vi "Sending Modulated Audio.vi"() -> ()   [LabVIEW 2019]
doc: "This application reads the selected audio file from its media storage. The audio is outputed through the Emona Communications Board for its modulation. After being modulated, the signal is inputed once again into the application. The modulated signal is now displayed through the Modulated Signal Graph and also is being sent to the other target by communicating with a TCP protocol."
uses:
  <vilib>/myRIO/Instrument Drivers/Onboard IO/AI Continuous/typedefs/AI Continuous Reference.ctl
  <vilib>/myRIO/Common/Instrument Driver Framework/Utilities/typedefs/myRIO Generic Hardware Reference.ctl
  <vilib>/myRIO/Common/Instrument Driver Framework/Utilities/typedefs/Hardware Version Enum.ctl
  <vilib>/myRIO/Common/Instrument Driver Framework/Utilities/typedefs/myRIO v1.0 Reference.ctl
  <vilib>/myRIO/Common/Instrument Driver Framework/Utilities/typedefs/Generic FPGA Reference.ctl
  <vilib>/myRIO/Common/Instrument Driver Framework/ELVIS III v1.0/AI Continuous/typedefs/AI Continuous Channels List.ctl
  <vilib>/myRIO/Common/Instrument Driver Framework/ELVIS III v1.0/AI Continuous/typedefs/ELVIS III v1.0 AI Continuous Channels Enum.ctl
  <vilib>/myRIO/Common/Instrument Driver Framework/Utilities/typedefs/Analog Scaling Constants.ctl
  <vilib>/userDefined/High Color/nirio_resource_hc.ctl
  <vilib>/myRIO/Instrument Drivers/Onboard IO/AO Continuous/typedefs/AO Continuous Reference.ctl
  <vilib>/myRIO/Common/Instrument Driver Framework/ELVIS III v1.0/AO Continuous/typedefs/AO Continuous Channels List.ctl
  <vilib>/myRIO/Common/Instrument Driver Framework/ELVIS III v1.0/AO Continuous/typedefs/ELVIS III v1.0 AO Continuous Channels Enum.ctl
  <vilib>/myRIO/Common/Instrument Driver Framework/ELVIS III v1.0/AO Continuous/typedefs/AO Continuous Channel Info.ctl
  <vilib>/myRIO/Instrument Drivers/Onboard IO/AO/typedefs/AO Reference.ctl
  <vilib>/myRIO/Common/Instrument Driver Framework/myRIO v1.0/AO/typedefs/AO Channels List.ctl
  <vilib>/myRIO/Common/Instrument Driver Framework/myRIO v1.0/AO/typedefs/AO Channels Enum.ctl
  <vilib>/myRIO/Common/Instrument Driver Framework/Utilities/typedefs/Analog Scaling Constants List.ctl
  <vilib>/myRIO/Common/Instrument Driver Framework/ELVIS III v1.0/AI Continuous/vis/ELVIS III v1.1 Open AI (Continuous).vi
  <vilib>/myRIO/Common/Instrument Driver Framework/ELVIS III v1.0/AO Continuous/vis/ELVIS III v1.1 Open AO (Continuous).vi
  <vilib>/myRIO/Common/Instrument Driver Framework/ELVIS III v1.0/AO/vis/ELVIS III v1.1 Open AO.vi
  <vilib>/myRIO/Common/Instrument Driver Framework/Utilities/vis/Validate Channels.vi
  <vilib>/myRIO/Common/Instrument Driver Framework/ELVIS III v1.0/AI Continuous/vis/ELVIS III v1.0 Reserve AI Continuous.vi
  <vilib>/myRIO/Common/Instrument Driver Framework/ELVIS III v1.0/AO Continuous/vis/ELVIS III v1.0 Reserve AO Continuous.vi
  <vilib>/myRIO/Common/Instrument Driver Framework/ELVIS III v1.0/AO/vis/ELVIS III v1.0 Reserve AO.vi
  <vilib>/myRIO/Common/Instrument Driver Framework/ELVIS III v1.0/AO Continuous/vis/ELVIS III v1.1 Close AO Continuous.vi
  <vilib>/myRIO/Common/Instrument Driver Framework/ELVIS III v1.0/AO/vis/ELVIS III v1.0 Close AO.vi
  <vilib>/myRIO/Common/Instrument Driver Framework/ELVIS III v1.0/AI Continuous/vis/ELVIS III v1.0 Close AI Continuous.vi
  <vilib>/myRIO/Common/Instrument Driver Framework/myRIO v1.0/UART/vis/myRIO v1.0 Close UART.vi
  <vilib>/myRIO/Common/Instrument Driver Framework/ELVIS III v1.0/AI Continuous/vis/ELVIS III v1.0 Build MUX Configuration AI Continuous.vi
  <vilib>/myRIO/Common/Instrument Driver Framework/ELVIS III v1.0/AO Continuous/vis/ELVIS III v1.0 Build MUX Configuration AO Continuous.vi
  <vilib>/myRIO/Common/Instrument Driver Framework/ELVIS III v1.0/AO/vis/ELVIS III v1.0 Build MUX Configuration AO.vi
  <vilib>/myRIO/Common/Instrument Driver Framework/ELVIS III v1.0/AO Continuous/vis/ELVIS III v1.0 Unreserve AO Continuous.vi
  <vilib>/myRIO/Common/Instrument Driver Framework/ELVIS III v1.0/AO/vis/ELVIS III v1.0 Unreserve AO.vi
  <vilib>/myRIO/Common/Instrument Driver Framework/ELVIS III v1.0/AI Continuous/vis/ELVIS III v1.0 Unreserve AI Continuous.vi
  <vilib>/Utility/VariantDataType/GetNumericInfo.vi
  <vilib>/Utility/error.llb/Error Cluster From Error Code.vi
  <vilib>/myRIO/Common/Instrument Driver Framework/ELVIS III v1.0/ELVIS III v1.1 Open.vi
  <vilib>/myRIO/Common/Instrument Driver Framework/ELVIS III v1.0/Resource Manager/vis/ELVIS III v1.0 Reserve Channel List.vi
  <vilib>/myRIO/Common/Instrument Driver Framework/myRIO v1.0/myRIO v1.0 Close.vi
  <vilib>/myRIO/Common/Instrument Driver Framework/ELVIS III v1.0/Resource Manager/vis/ELVIS III v1.0 Configure DMAs.vi
  <vilib>/myRIO/Common/Instrument Driver Framework/ELVIS III v1.0/AO Continuous/vis/ELVIS III v1.1 Stop AO Continuous.vi
  <vilib>/myRIO/Common/Instrument Driver Framework/ELVIS III v1.0/Resource Manager/vis/ELVIS III v1.0 Coerce AI Scaling.vi
  <vilib>/myRIO/Common/Instrument Driver Framework/ELVIS III v1.0/AI Continuous/vis/ELVIS III v1.1 Stop AI Continuous.vi
  <vilib>/myRIO/Common/Instrument Driver Framework/ELVIS III v1.0/AI Continuous/vis/ELVIS III v1.1 Start AI Continuous.vi
  <vilib>/myRIO/Common/Instrument Driver Framework/ELVIS III v1.0/AO Continuous/vis/ELVIS III v1.0 AO Continuous Write.vi
  <vilib>/myRIO/Common/Instrument Driver Framework/ELVIS III v1.0/AO/vis/ELVIS III v1.0 Write AO.vi
  <vilib>/myRIO/Common/Instrument Driver Framework/ELVIS III v1.0/AO Continuous/vis/ELVIS III v1.1 Start AO Continuous.vi
  <vilib>/myRIO/Common/Instrument Driver Framework/ELVIS III v1.0/AI Continuous/vis/ELVIS III v1.0 AI Continuous Read.vi
  <vilib>/myRIO/Common/Instrument Driver Framework/ELVIS III v1.0/Resource Manager/vis/ELVIS III v1.0 Unreserve Channel List.vi
  <vilib>/myRIO/Common/Instrument Driver Framework/Utilities/vis/FPGA Ref Manager.vi
  <vilib>/myRIO/Common/Instrument Driver Framework/ELVIS III v1.0/ELVIS III v1.0 Reset FPGA.vi
  <vilib>/myRIO/Common/Instrument Driver Framework/myRIO v1.0/IRQ/vis/myRIO v1.0 IRQ Info FGV.vi
  <vilib>/myRIO/Common/Instrument Driver Framework/myRIO v1.0/IRQ/vis/myRIO v1.0 Timer IRQ Info FGV.vi
  <vilib>/myRIO/Common/Instrument Driver Framework/myRIO v1.0/IRQ/vis/myRIO v1.0 ISR Agent.vi
  <vilib>/myRIO/Instrument Drivers/Utilities/vis/Reset Index.vi
  <vilib>/myRIO/Common/Instrument Driver Framework/myRIO v1.0/Resource Manager/vis/myRIO v1.0 Block Write Resource Manager.vi
  <vilib>/myRIO/Instrument Drivers/Onboard IO/AO/vis/myRIO AO Open.xnode
  <vilib>/myRIO/Instrument Drivers/Onboard IO/AO Continuous/vis/myRIO AO Continuous Open.xnode
  <vilib>/myRIO/Instrument Drivers/Onboard IO/AI Continuous/vis/myRIO AI Continuous Open.xnode
  <vilib>/myRIO/Instrument Drivers/Utilities/Utilities.lvlib
  <vilib>/myRIO/Instrument Drivers/Onboard IO/AO/AO.lvlib
  <vilib>/myRIO/Instrument Drivers/Onboard IO/AO Continuous/AO Continuous.lvlib
  <vilib>/myRIO/Instrument Drivers/Onboard IO/AI Continuous/AI Continuous.lvlib
panel:
  in  "Stop":bool
  in  "Select Audio":u16(ring) items=["ABBA- Dancing Queen.mp3", "Frank Sinatra - Fly Me To The Moon.mp3", "Gotye - Somebody That I Used To Know.mp3", "Mozart - Eine Kleine Nachtmusik.mp3"]
  in  "Address":string caption="Demodulator IP Address"
  out "Message":dbl[](graph) caption="Message History"
  in  "Offset":dbl=2.0
  out "Modulated Signal":dbl[](graph)
  out "error out":errorcluster
  in  "LocalStop":bool
  # "Sending and Modulating Audio"
  # "Explanation:\nThis application reads the selected audio file from its media storage. The audio is outputed through the Emona Communications Board for its modulation. After being modulated, the signal is inputed once again into the application. The modulated signal is now displayed through the Modulated Signal Graph and also is being sent to the other target by communicating with a TCP protocol.\n \nInstructions:\nAlways run the Receiving Modulated Audio VI before running this one. Remember to introduce the Demodulator IP Address into the control below. Check the instructions on the other VI for more information."
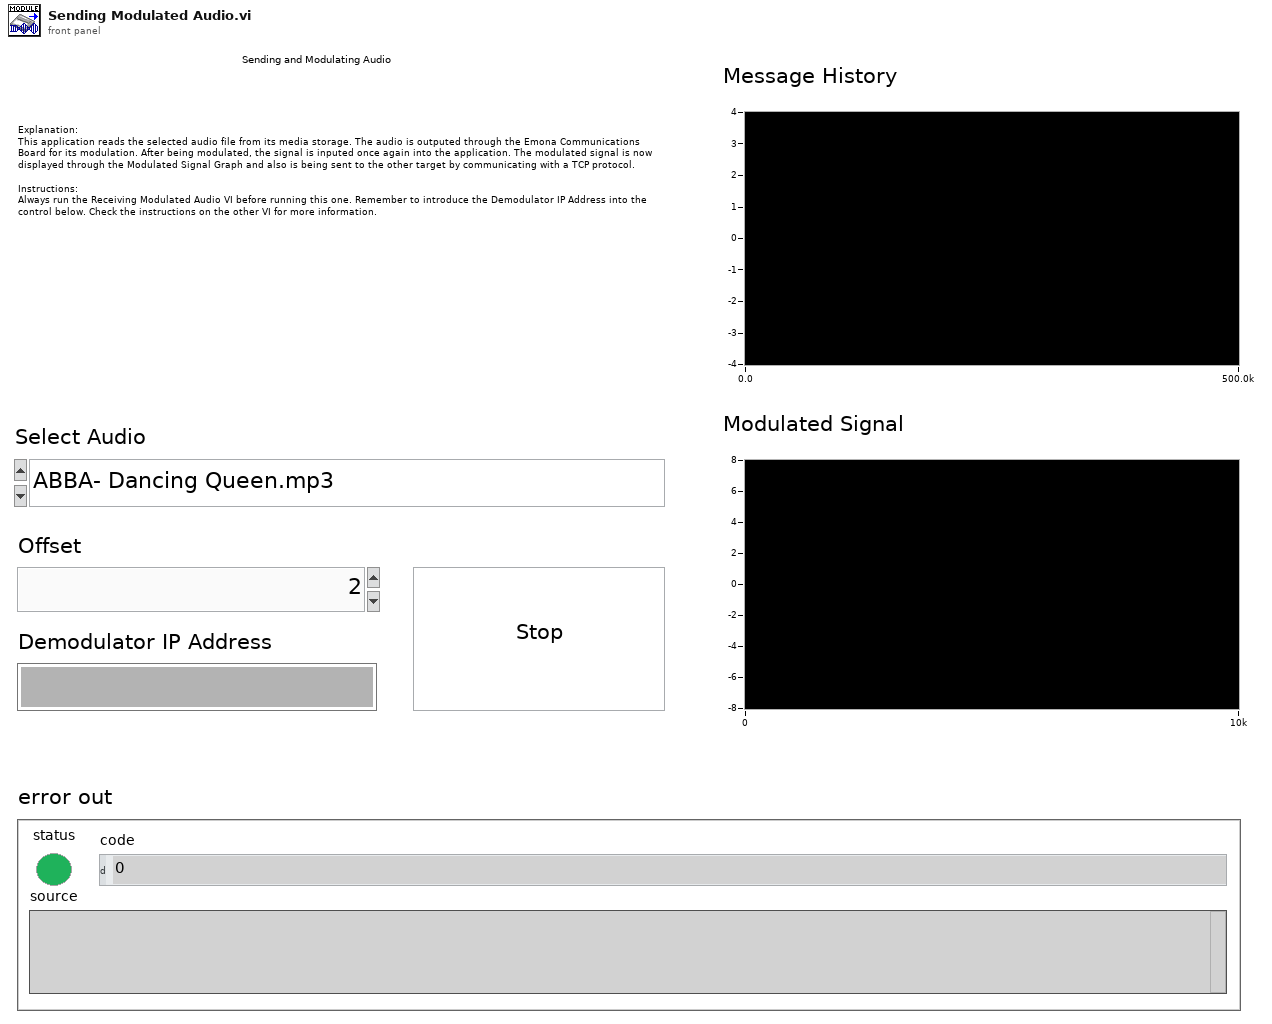
[diagram p1: front panel]
types:
  T1 = enum16{"open", "replace", "create", "open or create", "replace or create", "replace or create with confirmation"}
  T2 = typedef "AI Continuous.lvlib/AI Continuous Reference.ctl" = cluster{"myRIO Reference":T3, "AI (Continuous) Channels List":T7, "AI (Continuous) Scaling Constants List":T9[], "Bank Count":u8[]}
  T3 = typedef "myRIO Generic Hardware Reference.ctl" = cluster{"myRIO Model":T4, "myRIO Hardware Reference":T5}
  T4 = typedef "Hardware Version Enum.ctl" = enum16{"Unknown", "myRIO-1900", "myRIO-1950", "roboRIO", "NI ELVIS RIO CM", "ELVIS III"}
  T5 = typedef "myRIO v1.0 Reference.ctl" = cluster{"Generic FPGA Reference":T6, "Allow multiple opens":bool}
  T6 = typedef "Generic FPGA Reference.ctl" = refnum<k20>
  T7 = typedef "AI Continuous Channels List.ctl" = T8[]
  T8 = typedef "ELVIS III v1.0 AI Continuous Channels Enum.ctl" = enum16{"Not Connected", "A/AI0 (Continuous)", "A/AI1 (Continuous)", "A/AI2 (Continuous)", "A/AI3 (Continuous)", "A/AI4 (Continuous)", "A/AI5 (Continuous)", "A/AI6 (Continuous)", "A/AI7 (Continuous)", "A/AI0 (DIFF Continuous)", "A/AI1 (DIFF Continuous)", "A/AI2 (DIFF Continuous)", "A/AI3 (DIFF Continuous)", "B/AI0 (Continuous)", "B/AI1 (Continuous)", "B/AI2 (Continuous)", "B/AI3 (Continuous)", "B/AI4 (Continuous)", "B/AI5 (Continuous)", "B/AI6 (Continuous)", "B/AI7 (Continuous)", "B/AI0 (DIFF Continuous)", "B/AI1 (DIFF Continuous)", "B/AI2 (DIFF Continuous)", "B/AI3 (DIFF Continuous)"}
  T9 = typedef "Analog Scaling Constants.ctl" = cluster{"LSB Weight (Volts)":dbl, "Offset (Volts)":dbl, "Signed?":bool}
  T10 = typedef "AO Continuous.lvlib/AO Continuous Reference.ctl" = cluster{"myRIO Reference":T3, "AO (Continuous) Channels List":T11, "Channel Info":T13}
  T11 = typedef "AO Continuous Channels List.ctl" = T12[]
  T12 = typedef "ELVIS III v1.0 AO Continuous Channels Enum.ctl" = enum16{"Not Connected", "A/AO0 (Continuous)", "A/AO1 (Continuous)", "B/AO0 (Continuous)", "B/AO1 (Continuous)"}
  T13 = typedef "AO Continuous Channel Info.ctl" = cluster{"Channel Bitmask":u8[], "Channel Index":i32[], "Channel Number":u8}
  T14 = typedef "AO.lvlib/AO Reference.ctl" = cluster{"myRIO Reference":T3, "AO Channel List":T15, "AO Scaling Constant List":T17}
  T15 = typedef "AO Channels List.ctl" = T16[]
  T16 = typedef "AO Channels Enum.ctl" = enum16{"Not Connected", "AudioOut/Left", "AudioOut/Right", "C/AO0", "C/AO1", "A/AO0", "A/AO1", "B/AO0", "B/AO1"}
  T17 = typedef "Analog Scaling Constants List.ctl" = T9[]
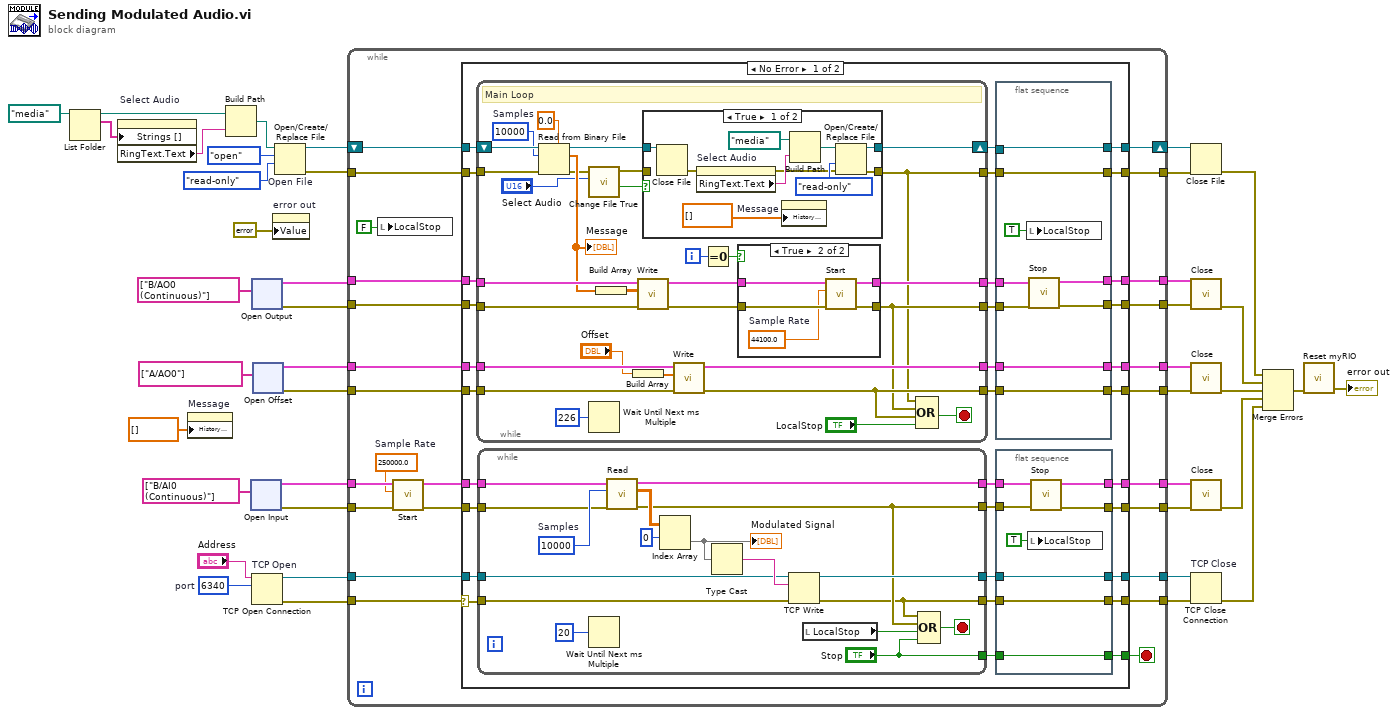
[diagram p0: block diagram]
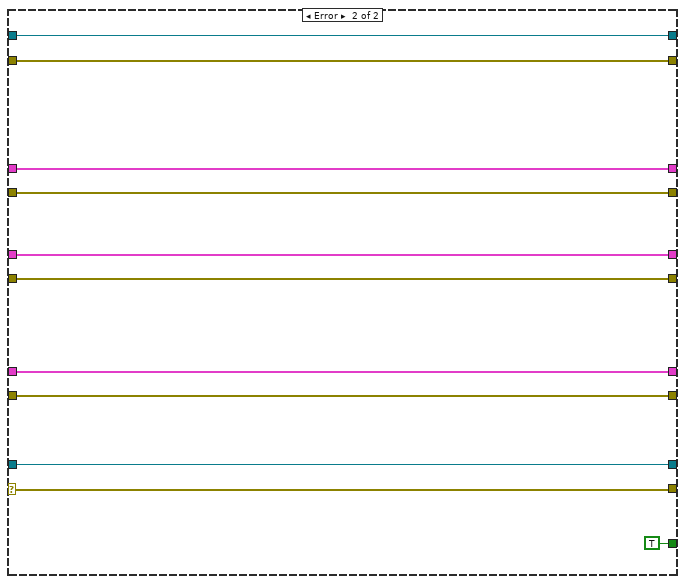
[diagram p4: hidden frame]
diagram:
  w17 = u16 6340  # port
  n1 = List Folder(path=path "/media") -> (path out=w10:path, filenames=w11:string[])  [unwired: 3 in, 2 out]
  n2 = property on="Select Audio" class="Ring (strict)"("Strings []"=w11) -> ("RingText.Text"=w9:string)  [unwired: 2 in, 2 out]
  n3 = property on="Message" class="WFChart (strict)"("History Data"=dbl[] []) -> ()  [unwired: 2 in, 2 out]
  n4 = Build Path(base path=w10, name or relative path=w9) -> (appended path=w13:path)
  n5 = xnode "Open Input"("Channel Names"=tag[] ["B/AI0 (Continuous)"]) -> ("error out"=w23:errorcluster, "AI (Continuous) Ref Out"=w22:T2)  [unwired: 3 in]
  n6 = xnode "Open Output"("Channel Names"=tag[] ["B/AO0 (Continuous)"]) -> ("error out"=w35:errorcluster, "AO (Continuous) Ref Out"=w36:T10)  [unwired: 1 in]
  n7 = TCP Open Connection "TCP Open"(address="Address", remote port or service name=w17) -> (connection ID=w25:refnum<k5>, error out=w24:errorcluster)  [unwired: 3 in]
  n8 = xnode "Open Offset"("Channel Names"=tag[] ["A/AO0"]) -> ("error out"=w40:errorcluster, "AO Ref Out"=w41:T14)  [unwired: 2 in]
  n9 = property on="error out" class="Clust (strict)"("Value"=errorcluster {"status"=FALSE, "code"=0, "source"=""} ("error constant")) -> ()  [unwired: 2 in, 2 out]
  n10 = Open/Create/Replace File "Open File"(file path (use dialog)=w13, operation (0:open)=T1."open", access (0:read/write)=enum16{"read/write", "read-only", "write-only"}."read-only") -> (refnum out=w38:refnum<file>, error out=w37:errorcluster)  [unwired: 3 in, 1 out]
  n11 = while {
    shift-right: [w57] -> w32
    shift-left: w38 -> [w63]
    tunnel: w24 -> [w43]
    tunnel: [w51] -> w26
    tunnel: w25 -> [w50]
    tunnel: [w52] -> w27
    tunnel: w23 -> [w49]
    tunnel: [w56] -> w31
    tunnel: w22 -> [w48]
    tunnel: [w55] -> w30
    tunnel: w40 -> [w65]
    tunnel: [w64] -> w39
    tunnel: w41 -> [w66]
    tunnel: [w59] -> w34
    tunnel: w35 -> [w60]
    tunnel: [w54] -> w29
    tunnel: w36 -> [w61]
    tunnel: [w53] -> w28
    tunnel: w37 -> [w62]
    tunnel: [w58] -> w33
    stop <- w42 stop-if-true
    w47 = 250000.0  # Sample Rate
    n12 = local write "LocalStop"(FALSE ("Stop")) -> ()
    n13 = call <vilib>:"Start.vi"("error in (no error)"=w49, "Sample Rate"=w47, "AI (Continuous) Ref In"=w48) -> ("error out"=w45:errorcluster, "AI (Continuous) Ref Out"=w46:T2)  [unwired: 7 in]
    n14 = case shown="No Error" w43 {
      selector: w43 -> [w69 w190]
      tunnel: w66 -> [w98 w186]
      tunnel: w65 -> [w97 w187]
      tunnel: [w96 w187] -> w64
      tunnel: w63 -> [w95 w182]
      tunnel: w62 -> [w94 w183]
      tunnel: w61 -> [w93 w184]
      tunnel: w60 -> [w92 w185]
      tunnel: [w91 w186] -> w59
      tunnel: [w90 w183] -> w58
      tunnel: [w89 w182] -> w57
      tunnel: [w88 w189] -> w56
      tunnel: [w87 w188] -> w55
      tunnel: [w86 w185] -> w54
      tunnel: [w85 w184] -> w53
      tunnel: [w84 w191] -> w52
      tunnel: [w83 w190] -> w51
      tunnel: w50 -> [w82 w191]
      tunnel: w46 -> [w71 w188]
      tunnel: w45 -> [w70 w189]
      tunnel: [w67 TRUE ("Stop")] -> w42
      frame No Error {
        n15 = while {
          tunnel: w98 -> [w162]
          tunnel: w97 -> [w161]
          tunnel: [w158] -> w80
          tunnel: [w157] -> w81
          tunnel: w94 -> [w155]
          tunnel: [w139] -> w77
          tunnel: w92 -> [w146]
          tunnel: [w144] -> w79
          tunnel: w93 -> [w147]
          tunnel: [w145] -> w78
          shift-right: [w140] -> w76
          shift-left: w95 -> [w156]
          i -> [w148]
          stop <- w159 stop-if-true
          w152 = 10000  # Samples
          # "Main Loop"
          n16 = Read from Binary File(5:0.0, 8:w155, 10:w152, 11:w156) -> (0:w137:errorcluster, 2:w141:dbl[], 3:w138:refnum<file>)  [unwired: 2 in, 1 out]
          "Message" <- w141
          n17 = call "Change File True.vi"("error in"=w137, "Numeric in"="Select Audio") -> ("error out"=w136:errorcluster, "Change song?"=w135:bool)  [unwired: 6 in, 1 out]
          n18 = Wait Until Next ms Multiple(millisecond multiple=u32 226) -> ()  [unwired: 1 out]
          n19 = Build Array(w141) -> (w143:dbl[][])
          n20 = Build Array("Offset") -> (w142:dbl[])
          n21 = call <vilib>:"Write.vi"("error in (no error)"=w146, "Data To Write"=w143, "AO (Continuous) Ref In"=w147) -> ("error out"=w150:errorcluster, "AO (Continuous) Ref Out"=w151:T10)  [unwired: 7 in]
          n22 = case shown="True" w135 {
            tunnel: [w169 w173] -> w139
            tunnel: w138 -> [w171 w174]
            tunnel: [w170 w174] -> w140
            tunnel: w136 -> [_ w173]
            frame True {
              n23 = Close File(refnum=w171) -> (error out=w164:errorcluster)  [unwired: 1 in, 1 out]
              n24 = property on="Select Audio" class="Ring (strict)"(error in=w164) -> (error out=w163:errorcluster, "RingText.Text"=w165:string)  [unwired: 1 in, 1 out]
              n25 = property on="Message" class="WFChart (strict)"("History Data"=dbl[] []) -> ()  [unwired: 2 in, 2 out]
              n26 = Build Path(base path=path "/media" ("path"), name or relative path=w165) -> (appended path=w167:path)
              n27 = Open/Create/Replace File ("Open File")(file path (use dialog)=w167, error in=w163, access (0:read/write)=enum16{"read/write", "read-only", "write-only"}."read-only") -> (refnum out=w170:refnum<file>, error out=w169:errorcluster)  [unwired: 3 in, 1 out]
            }
            frame False {
            }
          }
          n28 = call <vilib>:"Write.vi"("error in (no error)"=w161, "Values"=w142, "AO Ref In"=w162) -> ("error out"=w157:errorcluster, "AO Ref Out"=w158:T14)  [unwired: 6 in]
          n29 = Equal To 0?(x=w148) -> (x = 0?=w149:bool)
          n30 = case shown="True" w149 {
            tunnel: w151 -> [w176 w181]
            tunnel: w150 -> [w175 w180]
            tunnel: [w176 w179] -> w145
            tunnel: [w175 w178] -> w144
            frame False {
            }
            frame True {
              w177 = 44100.0  # Sample Rate
              n31 = call <vilib>:"Start.vi"("error in (no error)"=w180, "Sample Rate"=w177, "AO (Continuous) Ref In"=w181) -> ("error out"=w178:errorcluster, "AO (Continuous) Ref Out"=w179:T10)  [unwired: 7 in]
            }
          }
          n32 = Compound Arithmetic op=OR(w139, w144, w157, "LocalStop") -> (w159:bool)
        }
        n33 = while {
          tunnel: [w127] -> w75
          tunnel: [w123] -> w74
          tunnel: w82 -> [w121]
          tunnel: w69 -> [w120]
          tunnel: [w124] -> w73
          tunnel: [w122] -> w72
          tunnel: w71 -> [w118]
          tunnel: w70 -> [w117]
          tunnel: ["Stop"] -> w68
          stop <- w131 stop-if-true
          w129 = u32 10000  # Samples
          n34 = Wait Until Next ms Multiple(millisecond multiple=u32 20) -> ()  [unwired: 1 out]
          n35 = call <vilib>:"Read.vi"("error in (no error)"=w117, "Number of Samples"=w129, "AI (Continuous) Ref In"=w118) -> ("error out"=w123:errorcluster, "Values"=w128:dbl[][], "AI (Continuous) Ref Out"=w127:T2)  [unwired: 6 in]
          n36 = Index Array(array=w128, index (row)=0) -> (element=w126:dbl[])  [unwired: 1 in]
          "Modulated Signal" <- w126
          n37 = Type Cast(x=w126) -> (*(type *) &x=w125:string)  [unwired: 1 out]
          n38 = TCP Write(connection ID=w121, data in=w125, error in (no error)=w120) -> (connection ID out=w124:refnum<k5>, error out=w122:errorcluster)  [unwired: 2 out]
          n39 = local read "LocalStop"() -> (w130:bool)
          n40 = Compound Arithmetic op=OR(w122, w123, w130, "Stop") -> (w131:bool)
        }
        n41 = flat-sequence {
          tunnel: w81 -> [w115]
          tunnel: [w115] -> w96
          tunnel: [w114] -> w91
          tunnel: w80 -> [w114]
          tunnel: w79 -> [w107]
          tunnel: w78 -> [w108]
          tunnel: [w113] -> w90
          tunnel: w77 -> [w113]
          tunnel: w76 -> [w112]
          tunnel: [w112] -> w89
          tunnel: [w110] -> w86
          tunnel: [w109] -> w85
          frame #0 {
            n42 = local write "LocalStop"(TRUE ("Stop")) -> ()
            n43 = call <vilib>:"Stop.vi"("error in (no error)"=w107, "AO (Continuous) Ref In"=w108) -> ("error out"=w110:errorcluster, "AO (Continuous) Ref Out"=w109:T10)  [unwired: 8 in]
          }
        }
        n44 = flat-sequence {
          tunnel: w75 -> [w103]
          tunnel: w74 -> [w102]
          tunnel: [w105] -> w88
          tunnel: [w104] -> w87
          tunnel: w73 -> [w101]
          tunnel: [w101] -> w84
          tunnel: [w100] -> w83
          tunnel: w72 -> [w100]
          tunnel: w68 -> [w99]
          tunnel: [w99] -> w67
          frame #0 {
            n45 = local write "LocalStop"(TRUE ("Stop")) -> ()
            n46 = call <vilib>:"Stop.vi"("error in (no error)"=w102, "AI (Continuous) Ref In"=w103) -> ("error out"=w105:errorcluster, "AI (Continuous) Ref Out"=w104:T2)  [unwired: 8 in]
          }
        }
      }
      frame Error {
      }
    }
  }
  n47 = Close File(refnum=w32, error in=w33) -> (error out=w5:errorcluster)  [unwired: 1 out]
  n48 = call <vilib>:"Close.vi"("error in (no error)"=w29, "AO (Continuous) Ref In"=w28) -> ("error out"=w4:errorcluster)  [unwired: 9 in]
  n49 = call <vilib>:"Close.vi"("error in (no error)"=w39, "AO Ref In"=w34) -> ("error out"=w6:errorcluster)  [unwired: 9 in]
  n50 = call <vilib>:"Close.vi"("error in (no error)"=w31, "AI (Continuous) Ref In"=w30) -> ("error out"=w2:errorcluster)  [unwired: 9 in]
  n51 = TCP Close Connection "TCP Close"(connection ID=w27, error in (no error)=w26) -> (error out=w3:errorcluster)  [unwired: 2 out]
  n52 = Merge Errors(w5, w4, w6, w2, w3) -> (w7:errorcluster)
  n53 = call <vilib>:"Reset myRIO.vi"("error in (no error)"=w7) -> ("error out"=→"error out":errorcluster)  [unwired: 10 in]
